vi "Search for User.vi"(0 "iUser Configuration Manager DVR":refnum<data-value>, 5 "Username":string, 11 "error in":errorcluster) -> (4 "dup iUser Configuration Manager DVR":refnum<data-value>, 6 "Found":bool, 15 "error out":errorcluster)   [LabVIEW 2017, in "User Configuration Manager.lvlib" / "By Ref.lvlib"]
uses:
  <vilib>/gpm_packages/@cs/user-manager/Source/User Configuration Manager Ref/By Ref.lvlib
  <vilib>/gpm_packages/@cs/user-manager/Source/iUser Configuration Manager/iUser Configuration Manager.lvclass
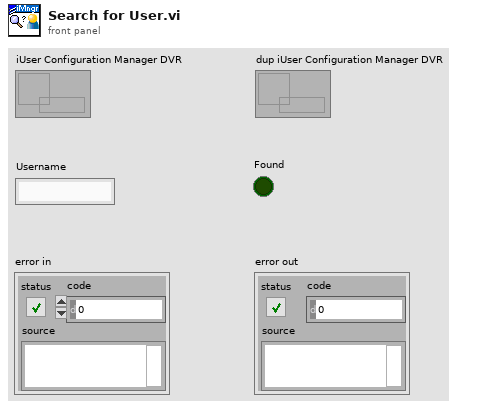
[diagram p1: front panel]
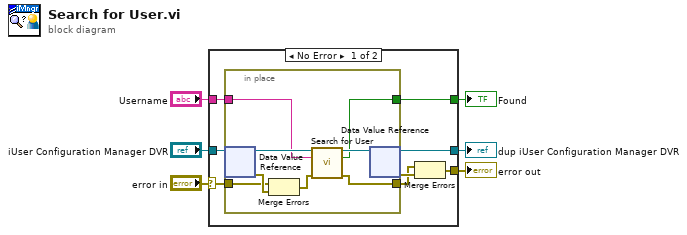
[diagram p0: block diagram]
diagram:
  n1 = case shown="No Error" "error in" {
    selector: "error in" -> [w12 w24]
    tunnel: "iUser Configuration Manager DVR" -> [w14 w23]
    tunnel: [w13 w24] -> w5
    tunnel: [w9 w23] -> w3
    tunnel: "Username" -> [w8 _]
    tunnel: [w7 _] -> w1
    frame No Error {
      n2 = in-place "IPES" {
        in-place-border: [w17] -> w10
        in-place-border: w12 -> [w21]
        in-place-border: w8 -> [w16]
        in-place-border: [w18] -> w7
        n3 = in-place-dvr #1(w14) -> (w20:refnum<class "iUser Configuration Manager.lvclass">, w22:errorcluster)
        n4 = Merge Errors(w21, w22) -> (w15:errorcluster)
        n5 = call-dynamic "Search for User.vi"("iUser Configuration Manager in"=w20, "Username"=w16, "error in (no error)"=w15) -> ("iUser Configuration Manager out"=w19:refnum<class "iUser Configuration Manager.lvclass">, "Found"=w18:bool, "error out"=w17:errorcluster)  [unwired: 10 in]
        n6 = in-place-dvr #1(w19) -> (w9:refnum<data-value>, w11:errorcluster)
      }
      n7 = Merge Errors(w10, w11) -> (w13:errorcluster)
    }
    frame Error {
    }
  }
  "error out" <- w5
  "dup iUser Configuration Manager DVR" <- w3
  "Found" <- w1
